vi "FG Timer.vi"(8 "error in (no error)":errorcluster, 10 "Target Duration (s)":dbl, 11 "Timer Commands":T1) -> (0 "error out":errorcluster, 1 "Elapsed Time":dbl, 2 "Done?":bool)   [LabVIEW 8.6]
doc: "A basic Functional Global timer that will return when a time has elapsed. Also returns time currently elapsed.\n\nStart Timer requires the Target Duration input and determines a target time of finishing.\nCheck Timer checks if the current time has reached that target time and returns True to Done? when it has."
uses:
  Controls/Timer Commands Enum.ctl
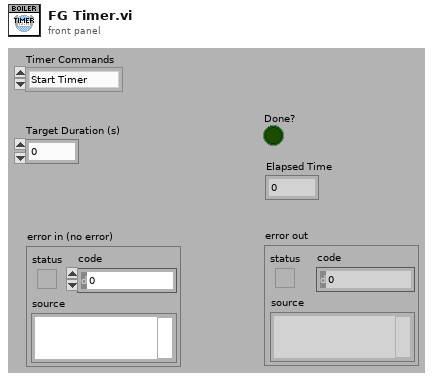
[diagram p1: front panel]
types:
  T1 = typedef "Timer Commands Enum.ctl" = enum16{"Start Timer", "Check Timer"}
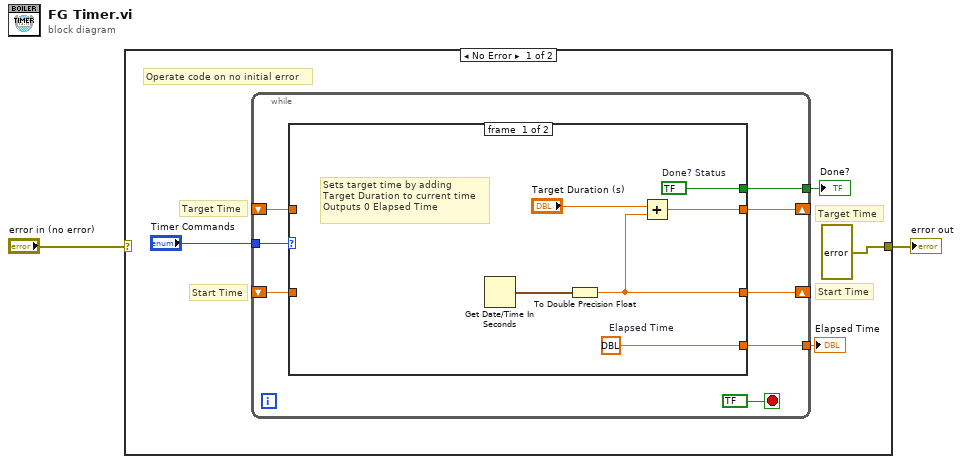
[diagram p0: block diagram]
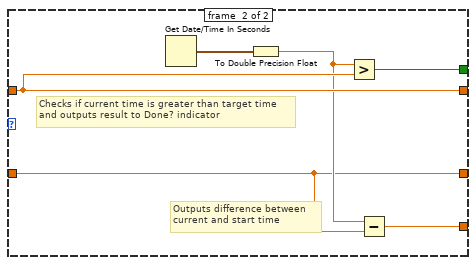
[diagram p2: hidden frame]
diagram:
  n1 = case shown="No Error" "error in (no error)" {
    selector: "error in (no error)" -> [_ w27]
    tunnel: [errorcluster ? ("error IO") w27] -> w1
    frame #0 {
      # "Start Time"
      # "Start Time"
      # "Target Time"
      # "Operate code on no initial error"
      # "Target Time"
      n2 = while {
        tunnel: "Timer Commands" -> [w13]
        shift-right: [w11] -> _
        shift-left: _ -> [w12]
        tunnel: [w10] -> w5
        shift-right: [w9] -> _
        shift-left: _ -> [w8]
        tunnel: [w7] -> w3
        stop <- bool ? stop-if-true
        n3 = case shown="\"Check Timer\"" w13 {
          tunnel: w12 -> [_ w24]
          tunnel: [w18 w24] -> w11
          tunnel: [w19 w25] -> w10
          tunnel: [w16 w22] -> w9
          tunnel: w8 -> [_ w22]
          tunnel: [w15 w21] -> w7
          frame #0 {
            w15 = dbl ?  # Elapsed Time
            w19 = bool ?  # Done? Status
            # "Sets target time by adding\nTarget Duration to current time\nOutputs 0 Elapsed Time"
            n4 = Get Date/Time In Seconds() -> (seconds since 1Jan1904=w20:timestamp)
            n5 = To Double Precision Float(number=w20) -> (double precision float=w16:dbl)
            n6 = Add(x="Target Duration (s)", y=w16) -> (x+y=w18:dbl)
          }
          frame #1 {
            # "Outputs difference between\ncurrent and start time"
            # "Checks if current time is greater than target time\nand outputs result to Done? indicator"
            n7 = Get Date/Time In Seconds() -> (seconds since 1Jan1904=w26:timestamp)
            n8 = To Double Precision Float(number=w26) -> (double precision float=w23:dbl)
            n9 = Greater?(x=w23, y=w24) -> (0:w25:bool)
            n10 = Subtract(x=w23, y=w22) -> (x-y=w21:dbl)
          }
        }
      }
      "Done?" <- w5
      "Elapsed Time" <- w3
    }
    frame #1 {
      # "Pass through error"
    }
  }
  "error out" <- w1
